vi "Manager+Read+Write.vi"() -> ()   [LabVIEW 2018]
uses:
  <vilib>/Analysis/Matrix/Datatypes/RealMatrix.ctl
  <instrlib>/Tektronix DMM40x0 Series/Tektronix DMM40x0 Series.lvlib
  LW/LIRA_toolbox.lvlib
  <vilib>/Analysis/Matrix/NI_Matrix.lvlib
panel:
  in  "Количество знаков\n после запятой величина 2":string="2"
  in  "Количество знаков\n после запятой величина 1":string="2"
  in  "Ширина строки\n(в символах) величина2":string="16"
  in  "Ширина строки \n(в символах) величина 1":string="16"
  out "Ошибка записи в файл":errorcluster
  out "Ошибка перключения":errorcluster
  in  "Задача":refnum<k21>="Generete_Termo_Dat"
  out "T1":T1(graph)
  in  "Function (0: DC Voltage)":u16(ring)=3 items=["DC Voltage", "AC Voltage", "2 - Wire Resistance", "4 - Wire Resistance", "DC Current", "AC Current", "Frequency", "Period", "Continuity", "Diode Checking", "Temperature", "Capacitance"]
  in  "Real Matrix":T2=[[0.0, 1.0, 0.0, 0.0], [0.0, 1.0, 0.0, 0.0], [0.0, 0.0, 0.0, 1.0], [0.0, 0.0, 0.0, 1.0], [0.0, 0.0, 1.0, 1.0], [0.0, 0.0, 1.0, 1.0]]
  in  "единицы измерения 2":string="C"
  in  "единицы измерения 1":string="Ом"
  in  "Сопротивление при нуле":dbl=60.0
  in  "alpha":dbl=0.00428
  in  "Измеряемая величина 2":string="T"
  in  "Измеряемая величина 1":string="R"
  out "Что следует из алгоритма":bool[](array[boolean])
  out "Array":bool[][](array[boolean])
  in  "Период перключения":dbl=2.0 caption="Delay Time (s)"
  in  "Название файла":string="TempData"
  in  "Путь к файлу с указанием\n на случайный txt файл":path=path "E:/Температурные датчики/Log/20250605_19_09_TempData.txt"
  in  "Количество датчиков":i32=4
  out "Ошибка прибора":errorcluster
  out "VISA resource name out":refnum<visa-resource-name>
  out "output array":dbl[](array[numeric]) format="%^_7e"
  in  "Serial Configuration":T3={"Baud Rate"=19200, "Parity"=0, "Data Bits"=8, "Stop Bits"=10, "Flow Control"=0} {"Flow Control" items=["None", "XON/XOFF", "RTS/CTS", "XON/XOFF & RTS/CTS", "DTR/DSR", "XON/XOFF & DTR/DSR"]; "Stop Bits" items=["1.0"=10, "1.5"=15, "2.0"=20]; "Data Bits" items=["7"=7, "8"=8]; "Parity" items=["None", "Odd", "Even", "Mark", "Space"]; "Baud Rate" items=["300"=300, "600"=600, "1200"=1200, "2400"=2400, "4800"=4800, "9600"=9600, "19200"=19200]}
  in  "VISA resource name":refnum<visa-resource-name>="COM5"
  in  "stop":bool
  # "Параметры для создания log файла"
  # "Схема включения каналов"
  # "Каждая колонка соответсвует определённому датчику\nКаждый ряд соответствует определённому реле"
  # "Параметры для расчёта температуры"
  # "Параметры процесса измерения"
  # "Подключение к измерительному прибору"
  # "Индикация для отадки"
  # "График температур"
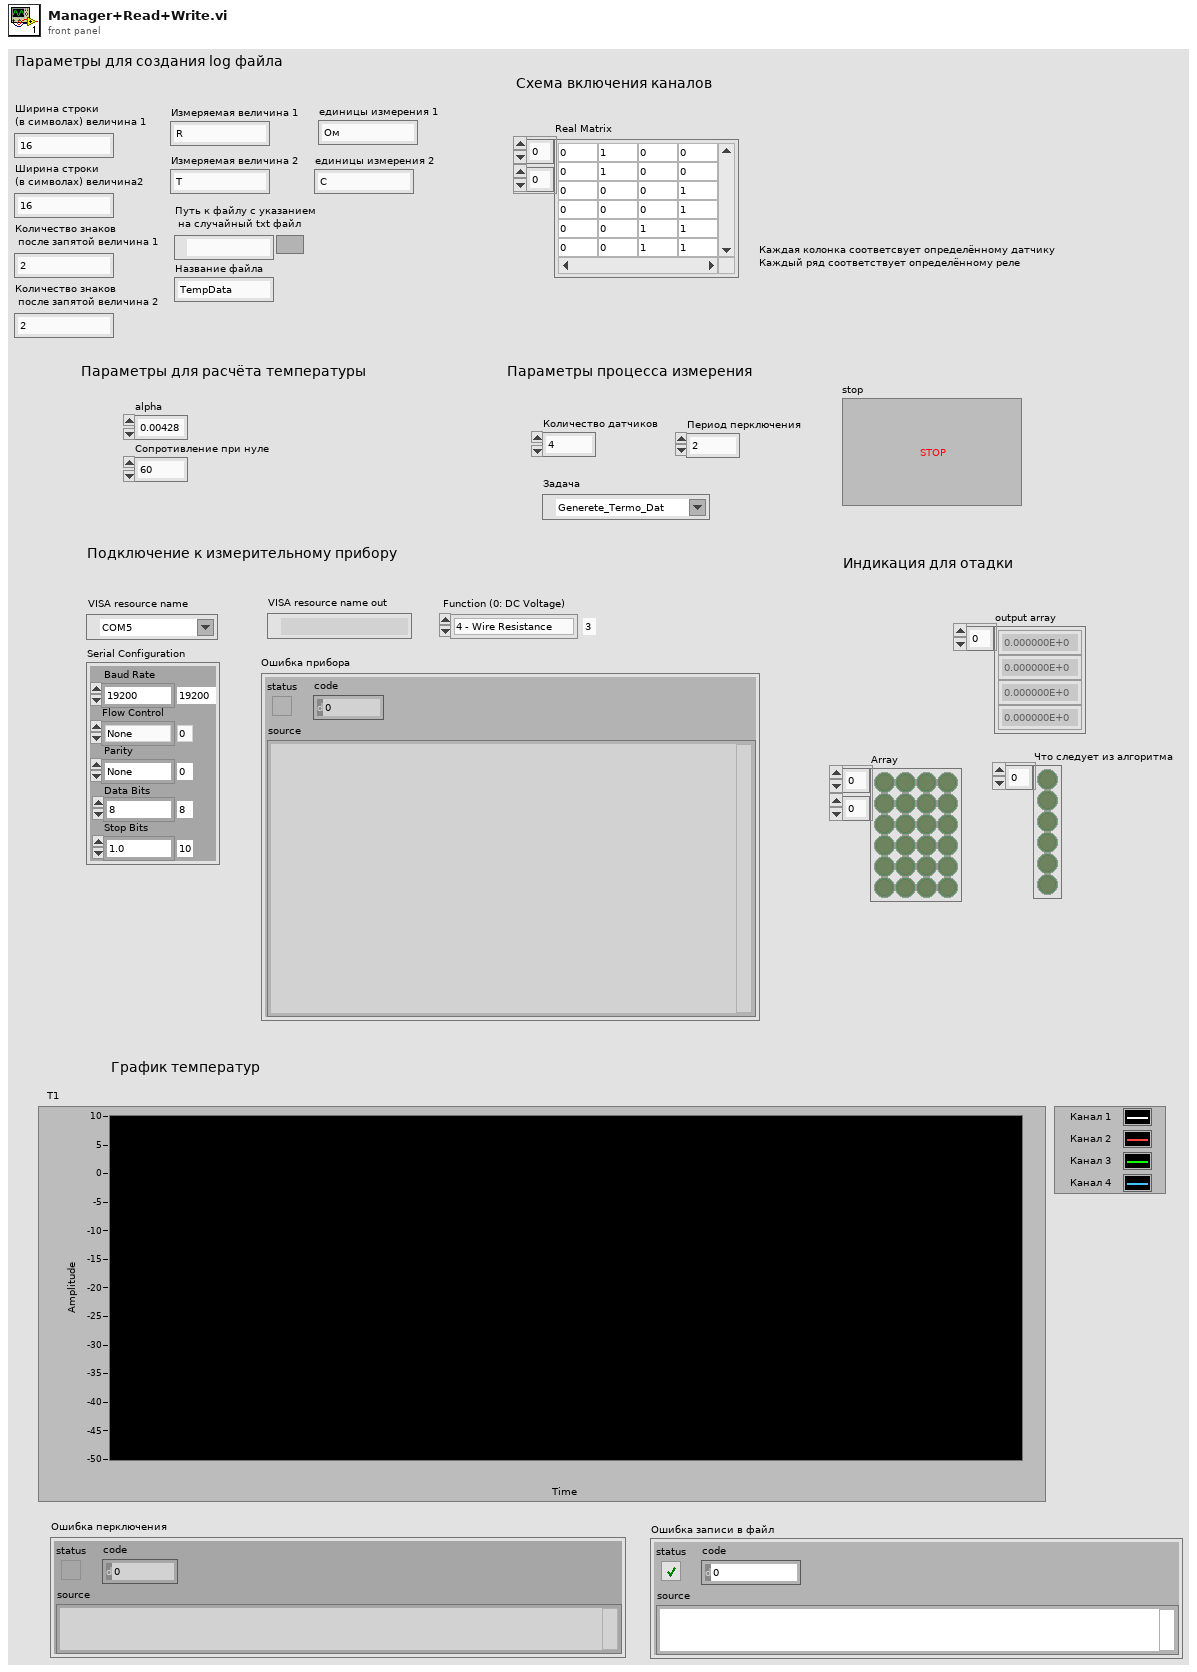
[diagram p1: front panel]
types:
  T1 = cluster{"Массив температур[0]":dbl, "Массив температур[1]":dbl, "Массив температур[2]":dbl, "Массив температур[3]":dbl, "Массив температур[4]":dbl, "Массив температур[5]":dbl, "Массив температур[6]":dbl, "Массив температур[7]":dbl, "Массив температур[8]":dbl}
  T2 = typedef "NI_Matrix.lvlib/RealMatrix.ctl" = dbl[][]
  T3 = cluster{"Baud Rate":u32, "Parity":u16, "Data Bits":u16, "Stop Bits":u16, "Flow Control":u16}
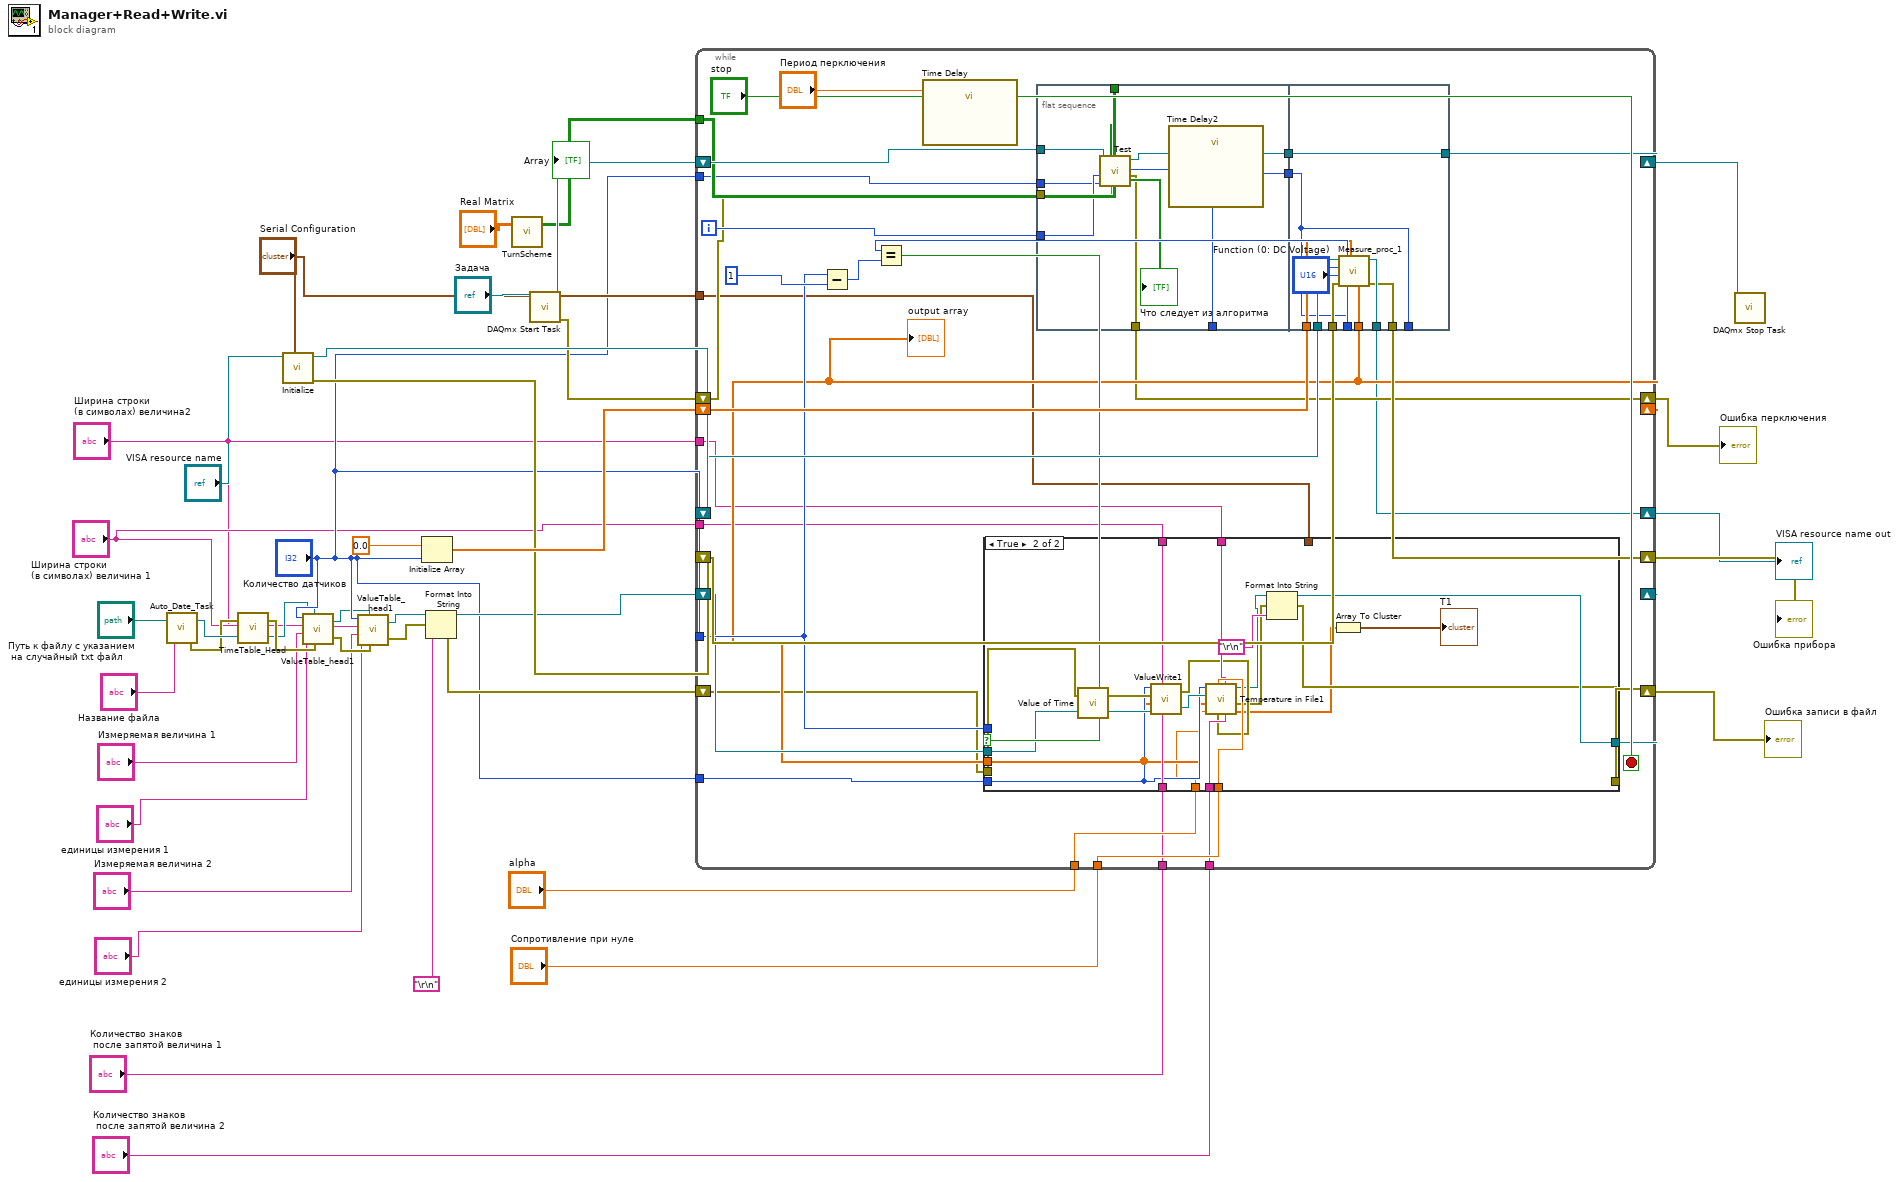
[diagram p0: block diagram]
diagram:
  n1 = call "Auto_Date_Task.vi"("Название файла"="Название файла", "Путь к файлу с указанием на случайный txt файл"="Путь к файлу с указанием\n на случайный txt файл") -> ("error out"=w19:errorcluster, "refnum out"=w25:refnum<file>)
  n2 = call "TimeTable_Head.vi"("input file"=w25, "error in"=w19) -> ("output file refnum"=w7:refnum<file>, "error out"=w15:errorcluster)
  n3 = call <instrlib>:"Initialize.vi"("Serial Configuration"="Serial Configuration", "VISA resource name"="VISA resource name") -> ("error out"=w35:errorcluster, "VISA resource name out"=w37:refnum<visa-resource-name>)  [unwired: 8 in]
  n4 = call "ValueTable_head1.vi"("error in 2"=w15, "Файл записи"=w7, "единицы измерения"="единицы измерения 1", "Измеряемая величина"="Измеряемая величина 1", "Ширина строки (в символах)"="Ширина строки \n(в символах) величина 1", "Количество датчиков"="Количество датчиков") -> ("error out"=w14:errorcluster, "Файл записи 2"=w6:refnum<file>)
  n5 = call "ValueTable_head1.vi"("error in 2"=w14, "Файл записи"=w6, "единицы измерения"="единицы измерения 2", "Измеряемая величина"="Измеряемая величина 2", "Ширина строки (в символах)"="Ширина строки\n(в символах) величина2", "Количество датчиков"="Количество датчиков") -> ("error out"=w13:errorcluster, "Файл записи 2"=w5:refnum<file>)
  n6 = Initialize Array(0.0 ("element"), "Количество датчиков") -> (w36:dbl[])
  n7 = Format Into String(initial string=w5, error in=w13, "\r\n") -> (resulting string=w28:refnum<file>, error out=w18:errorcluster)  [unwired: 1 in]
  n8 = call "TurnScheme.vi"("Real Matrix"="Real Matrix") -> ("Array"=w26:bool[][])  [unwired: 2 in]
  "Array" <- w26
  n9 = call <vilib>:"DAQmx Start Task.vi"("task/channels in"="Задача") -> ("task out"=w39:refnum<k21>, "error out"=w21:errorcluster)  [unwired: 13 in]
  n10 = while {
    shift-right: [w57] -> w40
    shift-left: w39 -> [w73]
    shift-right: [w68] -> w34
    shift-left: w35 -> [w69]
    tunnel: "Количество датчиков" -> [w61]
    shift-right: [w54] -> _
    shift-left: w36 -> [w67]
    shift-right: [w59] -> _
    shift-left: w28 -> [w60]
    shift-right: [w45] -> w32
    shift-left: w37 -> [w70]
    tunnel: w26 -> [w58]
    tunnel: "alpha" -> [w56]
    tunnel: "Сопротивление при нуле" -> [w55]
    tunnel: "Количество датчиков" -> [w52]
    tunnel: "Количество датчиков" -> [w51]
    shift-right: [w49] -> w20
    shift-left: w21 -> [w50]
    shift-right: [w47] -> w17
    shift-left: w18 -> [w48]
    tunnel: "Serial Configuration" -> [w46]
    tunnel: "Ширина строки \n(в символах) величина 1" -> [w44]
    tunnel: "Количество знаков\n после запятой величина 1" -> [w43]
    tunnel: "Ширина строки\n(в символах) величина2" -> [w42]
    tunnel: "Количество знаков\n после запятой величина 2" -> [w41]
    i -> [w53]
    stop <- "stop" stop-if-true
    n11 = Subtract(x=w61, y=1) -> (x-y=w64:i32)
    n12 = Equal?(x=w66, y=w64) -> (x = y?=w62:bool)
    n13 = call "Time Delay"("Delay Time (s)"="Период перключения") -> ()  [unwired: 10 in, 1 out]
    n14 = case shown="True" w62 {
      tunnel: w61 -> [_ _]
      tunnel: w54 -> [_ w86]
      tunnel: w60 -> [w76 w95]
      tunnel: [w76 w96] -> w59
      tunnel: w56 -> [_ w85]
      tunnel: w55 -> [_ w84]
      tunnel: w51 -> [_ w87]
      tunnel: w48 -> [w75 w94]
      tunnel: [w75 w93] -> w47
      tunnel: w46 -> [_ _]
      tunnel: w44 -> [_ w89]
      tunnel: w43 -> [_ w88]
      tunnel: w42 -> [_ w83]
      tunnel: w41 -> [_ w82]
      frame False {
      }
      frame True {
        n15 = call "Value of Time.vi"("input file"=w95, "error in"=w94) -> ("output file refnum"=w92:refnum<file>, "error out"=w91:errorcluster)
        n16 = call "ValueWrite1.vi"("Количество знаков после запятой"=w88, "Ширина строки (в символах)"=w89, "Файл с заголовком"=w92, "Массив с измерениями"=w86, "error in"=w91, "Количество датчиков"=w87) -> ("Файл с заголовком 2"=w90:refnum<file>, "error out"=w81:errorcluster)
        n17 = call "Temperature in File1.vi"("Количество знаков после запятой"=w82, "Ширина строки (в символах)"=w83, "error in"=w81, "Сопротивление при нуле"=w84, "Значение температурного коэффициента"=w85, "массив с сопротивлениями"=w86, "Файл"=w90, "Количество датчиков"=w87) -> ("Массив температур"=w79:dbl[], "error out"=w80:errorcluster, "Файл 2"=w77:refnum<file>)  [unwired: 1 in]
        n18 = Format Into String(initial string=w77, error in=w80, "\r\n") -> (resulting string=w96:refnum<file>, error out=w93:errorcluster)  [unwired: 1 in]
        n19 = Array To Cluster(array=w79) -> (cluster=→"T1":T1)
      }
    }
    n20 = flat-sequence {
      tunnel: w73 -> [w106]
      tunnel: [w105] -> w72
      tunnel: [w102] -> w71
      tunnel: w58 -> [w104]
      tunnel: [w102] -> _
      tunnel: w53 -> [w101]
      tunnel: w52 -> [w100]
      tunnel: w50 -> [w99]
      tunnel: [w98] -> w49
      tunnel: w72 -> [w108]
      tunnel: w71 -> [w109]
      tunnel: w70 -> [w115]
      tunnel: [w114] -> w45
      tunnel: w69 -> [w113]
      tunnel: [w112] -> w68
      tunnel: w67 -> [w111]
      tunnel: [w110] -> w54
      tunnel: [w109] -> _
      tunnel: [w109] -> w66
      tunnel: [w108] -> w57
      frame #0 {
        n21 = call "Test.vi"("error in"=w99, "array"=w104, "Количество датчиков"=w100, "Номер иттерации"=w101, "task/channels in"=w106) -> ("Индекс переключаемого канала"=w102:i32, "error out"=w98:errorcluster, "task out"=w105:refnum<k21>, "Что следует из алгоритма"=→"Что следует из алгоритма":bool[])  [unwired: 3 in]
        n22 = call "Time Delay2"() -> ()  [unwired: 11 in, 1 out]
      }
      frame #1 {
        n23 = call "Measure_proc_1.vi"("array"=w111, "error in (no error)"=w113, "Function (0: DC Voltage)"="Function (0: DC Voltage)", "Индекс записываемого канала"=w109, "VISA resource name"=w115) -> ("error out"=w112:errorcluster, "VISA resource name out"=w114:refnum<visa-resource-name>, "output array"=w110:dbl[])  [unwired: 4 in]
      }
    }
    "output array" <- w54
  }
  "VISA resource name out" <- w32
  "Ошибка прибора" <- w34
  "Ошибка перключения" <- w20
  "Ошибка записи в файл" <- w17
  n24 = call <vilib>:"DAQmx Stop Task.vi"("task/channels in"=w40) -> ()  [unwired: 13 in, 2 out]
